vi "Get ASI LED power.vi"(8 "error in":errorcluster, 11 "VISA resource in":refnum<visa-resource-name>) -> (0 "error out":errorcluster, 2 "LED power":i32, 3 "VISA resource name out":refnum<visa-resource-name>)   [LabVIEW 2018]
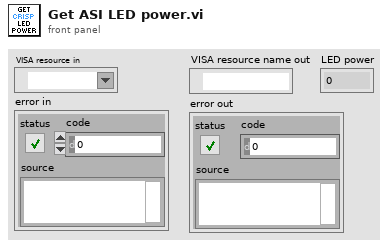
[diagram p1: front panel]
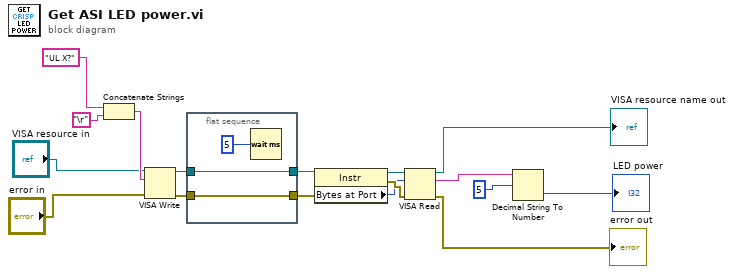
[diagram p0: block diagram]
diagram:
  n1 = Concatenate Strings("UL X?" ("write buffer"), "\r") -> (w17:string)
  n2 = VISA Write(VISA resource name="VISA resource in", write buffer=w17, error in (no error)="error in") -> (VISA resource name out=w10:refnum<visa-resource-name>, error out=w9:errorcluster)  [unwired: 1 out]
  n3 = flat-sequence {
    tunnel: [w20] -> w7
    tunnel: w10 -> [w20]
    tunnel: [w18] -> w8
    tunnel: w9 -> [w18]
    frame #0 {
      n4 = Wait (ms)(milliseconds to wait=u32 5) -> ()  [unwired: 1 out]
    }
  }
  n5 = property class="Instr"(reference=w7, error in=w8) -> (reference out=w11:refnum<visa-resource-name>, error out=w13:errorcluster, "Bytes at Port"=w12:u32)
  n6 = VISA Read(VISA resource name=w11, byte count=w12, error in (no error)=w13) -> (VISA resource name out=→"VISA resource name out":refnum<visa-resource-name>, read buffer=w3:string, error out=→"error out":errorcluster)  [unwired: 1 out]
  n7 = Decimal String To Number(string=w3, offset=5 ("offset (0)")) -> (number=→"LED power":i32)  [unwired: 1 in, 1 out]
